vi "OnErrorMessage Event Callback.vi"(4 "error in (no error)":refnum<user-event>, 5 "Event Data":cluster{"errCode":u32, "errString":string}, 6 "Control Ref":refnum<k24>, 7 "Event Common Data":T1) -> ()   [LabVIEW 2020, in "NI_VS MacroPlayerAPI.lvlib"]
uses:
  <vilib>/NI VeriStand/Execution/MacroPlayer/NI_VS MacroPlayerAPI.lvlib
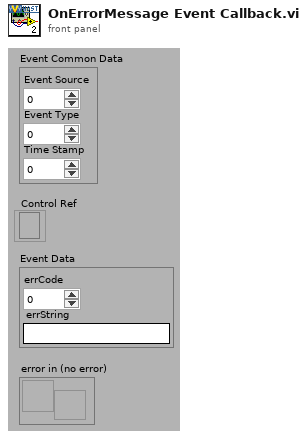
[diagram p1: front panel]
types:
  T1 = cluster{"Event Source":i32, "Event Type":u32, "Time Stamp":u32}
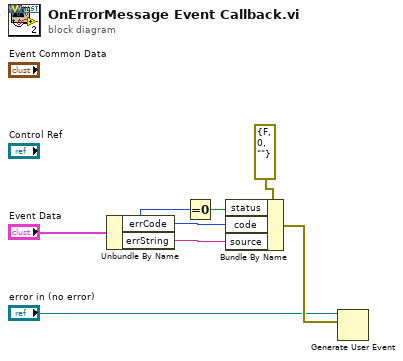
[diagram p0: block diagram]
diagram:
  n1 = Unbundle By Name("Event Data") -> ("errCode"=w4:u32, "errString"=w6:string)
  n2 = Equal To 0?(x=w4) -> (x = 0?=w5:bool)
  n3 = Bundle By Name(cluster=errorcluster {"status"=FALSE, "code"=0, "source"=""} ("Error"), "status"=w5, "code"=w4, "source"=w6) -> (w2:errorcluster)
  n4 = Generate User Event(user event="error in (no error)", event data cluster=w2) -> ()  [unwired: 2 in, 2 out]
